vi "Day07-1.vi"() -> ()   [LabVIEW 2021]
uses:
  f00bd700-c5e9-4b99-81d8-9b982d1785ce.vi
panel:
  out "Total Fuel Needed":i64
  out "input values":i64[](array[numeric])
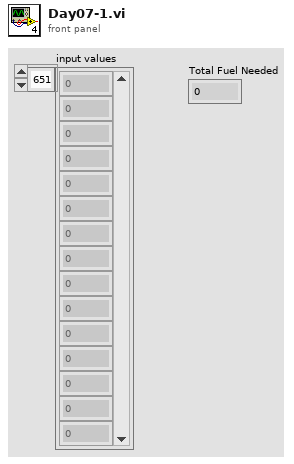
[diagram p1: front panel]
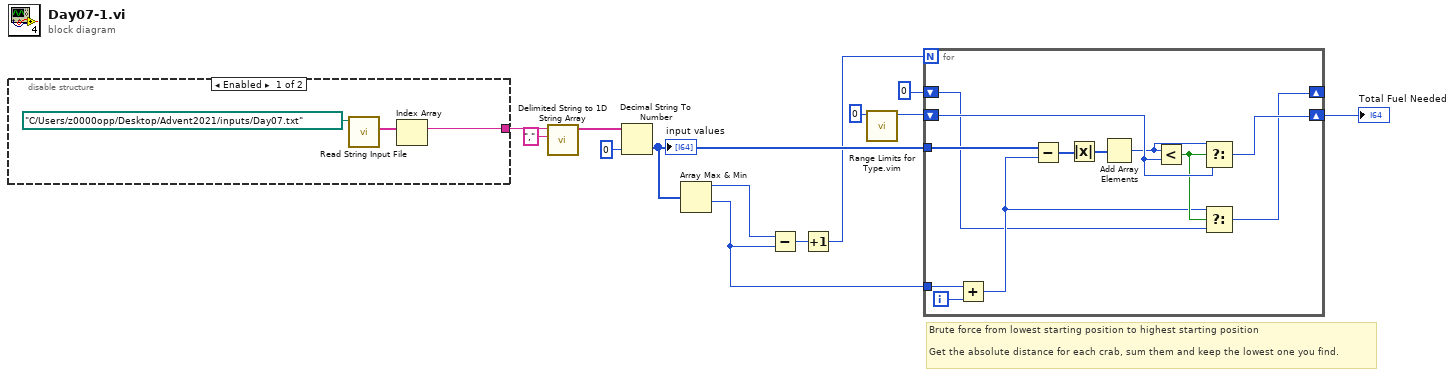
[diagram p0: block diagram]
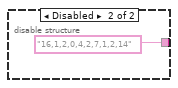
[diagram p2: hidden frame]
diagram:
  # "Brute force from lowest starting position to highest starting position\n\nGet the absolute distance for each crab, sum them and keep the lowest one you find."
  n1 = disable-structure shown="Enabled" {
    disable-tunnel: [w14 "16,1,2,0,4,2,7,1,2,14" ("String")] -> w10
    frame Enabled {
      n2 = call "Read String Input File.vi"("file path (dialog if empty)"=path "C:/Users/z0000opp/Desktop/Advent2021/inputs/Day07.txt") -> ("input values"=w15:string[])  [unwired: 10 in]
      n3 = Index Array(array=w15) -> (element=w14:string)  [unwired: 1 in]
    }
    frame Disabled {
    }
  }
  n4 = call <vilib>:"Delimited String to 1D String Array.vi"("delimiter"=",", "delimited string"=w10) -> ("string array"=w13:string[])  [unwired: 9 in]
  n5 = Decimal String To Number(string=w13, default (0L)=i64 0 ("default (0 I32)")) -> (number=w9:i64[])  [unwired: 1 in, 1 out]
  "input values" <- w9
  n6 = Array Max & Min(array=w9) -> (max value=w8:i64, min value=w5:i64)  [unwired: 2 out]
  n7 = Subtract(x=w8, y=w5) -> (x-y=w7:i64)
  n8 = Increment(x=w7) -> (x+1=w6:i64)
  n9 = call "Range Limits for Type.vim"("type"=0) -> ("maximum value for type"=w3:i32)  [unwired: 9 in, 1 out]
  n10 = for {
    N: w6 -> [_]
    tunnel: w9 -> [w27]
    tunnel: w5 -> [w28]
    shift-right: [w19] -> _
    shift-left: 0 -> [w18]
    shift-right: [w22] -> w1
    shift-left: w3 -> [w24]
    i -> [w29]
    n11 = Add(x=w28, y=w29) -> (x+y=w20:i64)
    n12 = Subtract(x=w27, y=w20) -> (x-y=w26:i64[])
    n13 = Absolute Value(x=w26) -> (abs(x)=w25:i64[])
    n14 = Add Array Elements(numeric array=w25) -> (sum=w23:i64)
    n15 = Less?(x=w23, y=w24) -> (x < y?=w21:bool)
    n16 = Select(t=w23, s=w21, f=w24) -> (s? t:f=w22:i64)
    n17 = Select(t=w20, s=w21, f=w18) -> (s? t:f=w19:i64)
  }
  "Total Fuel Needed" <- w1
